vi "freq_testing.vi"() -> ()   [LabVIEW 2015]
uses:
  <vilib>/Utility/file.llb/Read Delimited Spreadsheet (DBL).vi
panel:
  out "al  fitness":dbl[][](array[numeric])
  out "q4":dbl[](graph)
  out "q3":dbl[](graph)
  out "q2":dbl[](graph)
  out "q1":dbl[](graph)
  out "q0":dbl[](graph)
  out "q_output":dbl[](array[numeric])
  out "q diff":dbl[][](array[numeric])
  out "qfreq":dbl[](array[numeric])
  in  "qfreq path":path=path "D:/OneDrive/COURSES/LAB/2.LABVIEW_CODE/simulation/data/freqdata/qfreq.txt"
  out "length":i32
  out "qrls":dbl[](array[numeric])
  out "size(s)":i32[](array[numeric])
  in  "qrls path":path=path "D:/OneDrive/COURSES/LAB/2.LABVIEW_CODE/simulation/data/freqdata/qrls.txt"
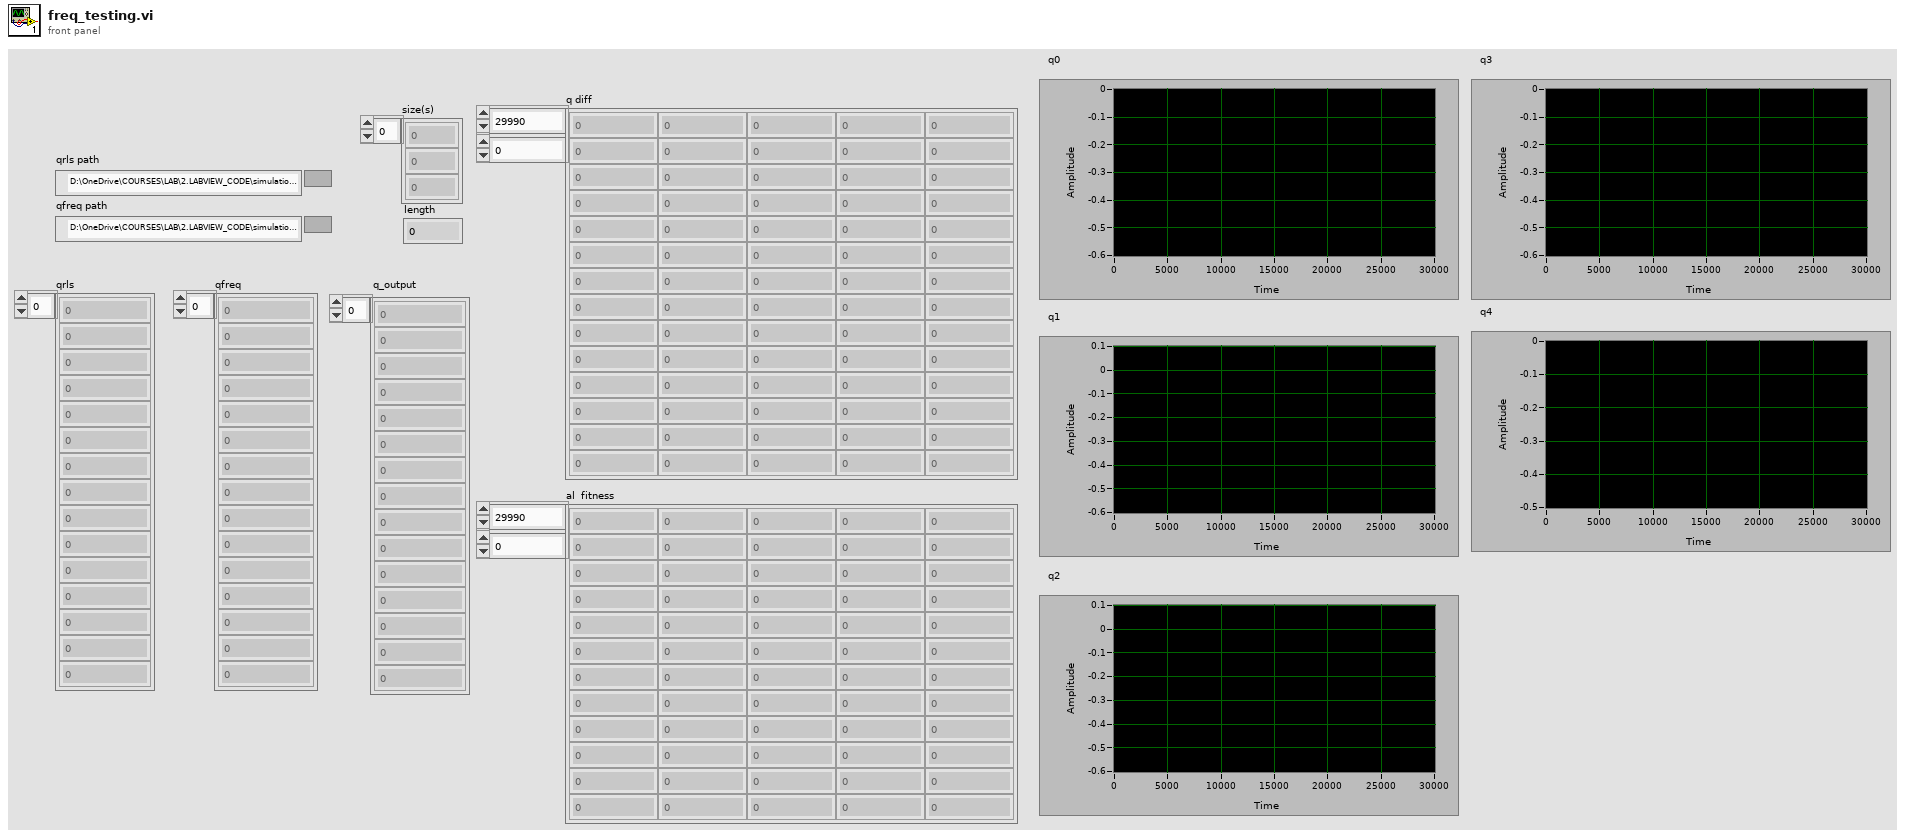
[diagram p1: front panel]
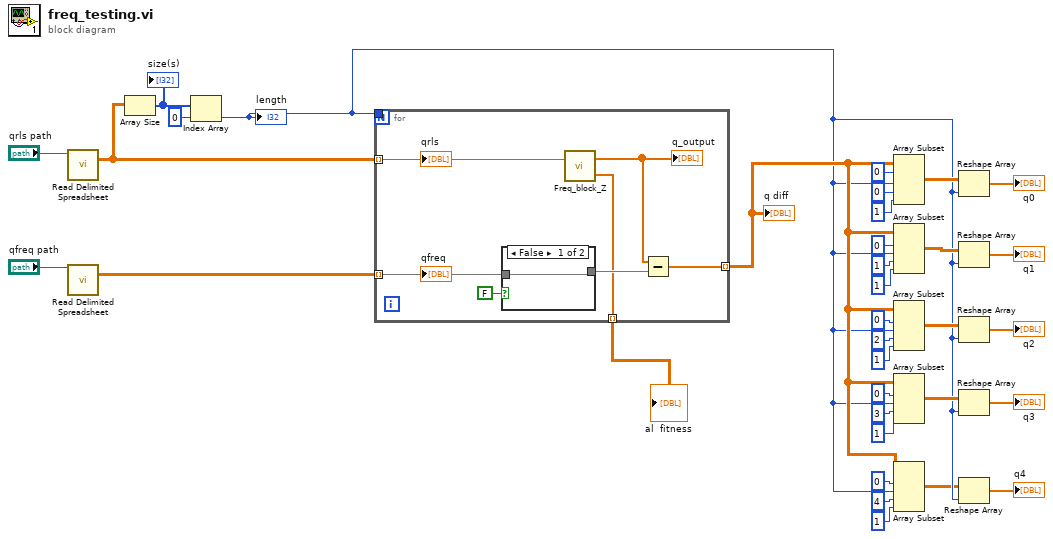
[diagram p0: block diagram]
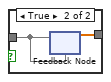
[diagram p2: hidden frame]
diagram:
  n1 = call-poly <vilib>:"Read Delimited Spreadsheet.vi"("file path (dialog if empty)"="qrls path") -> ("all rows"=w30:dbl[][])  [unwired: 9 in, 5 out]
  n2 = call-poly <vilib>:"Read Delimited Spreadsheet.vi"("file path (dialog if empty)"="qfreq path") -> ("all rows"=w29:dbl[][])  [unwired: 9 in, 5 out]
  n3 = Array Size(array=w30) -> (size(s)=w32:i32[])
  "size(s)" <- w32
  n4 = Index Array(array=w32, index=0) -> (element=w4:i32)
  "length" <- w4
  n5 = for {
    tunnel: w30 -> [w41] mode=indexing
    tunnel: w29 -> [w37] mode=indexing
    tunnel: [w39] -> w6 mode=indexing
    tunnel: w4 -> [_]
    tunnel: [w35] -> w1 mode=indexing
    n6 = case shown="False" FALSE {
      tunnel: [w42 w44] -> w38
      tunnel: w37 -> [w42 w43]
      frame False {
      }
      frame True {
        n7 = feedback #1(w43) -> (w44:dbl[])
        n8 = feedback-in #1(w43) -> ()
      }
    }
    n9 = call "Freq_block_Z.vi"("q_input"=w41) -> ("al  fitness"=w35:dbl[], "q_output"=w40:dbl[])  [unwired: 1 in]
    "q_output" <- w40
    n10 = Subtract(x=w40, y=w38) -> (x-y=w39:dbl[])
    "qrls" <- w41
    "qfreq" <- w37
  }
  "q diff" <- w6
  "al  fitness" <- w1
  n11 = Array Subset(array=w6, index (row)=0 ("index"), length (row)=w4, index (col)=0 ("index"), length (col)=1 ("length")) -> (w25:dbl[][])
  n12 = Array Subset(array=w6, index (row)=0 ("index"), length (row)=w4, index (col)=1 ("index"), length (col)=1 ("length")) -> (w19:dbl[][])
  n13 = Array Subset(array=w6, index (row)=0 ("index"), length (row)=w4, index (col)=2 ("index"), length (col)=1 ("length")) -> (w14:dbl[][])
  n14 = Array Subset(array=w6, index (row)=0 ("index"), length (row)=w4, index (col)=3 ("index"), length (col)=1 ("length")) -> (w9:dbl[][])
  n15 = Array Subset(array=w6, index (row)=0 ("index"), length (row)=w4, index (col)=4 ("index"), length (col)=1 ("length")) -> (w3:dbl[][])
  n16 = Reshape Array(w25, w4) -> (→"q0":dbl[])
  n17 = Reshape Array(w19, w4) -> (→"q1":dbl[])
  n18 = Reshape Array(w14, w4) -> (→"q2":dbl[])
  n19 = Reshape Array(w9, w4) -> (→"q3":dbl[])
  n20 = Reshape Array(w3, w4) -> (→"q4":dbl[])
